vi "rad_Button and Menu Status.vi"(9 "Manager Permissions":bool, 10 "App Image List":i32, 11 "Target List":i32[](array[numeric])) -> (0 "Retrieve AppImage":bool, 1 "Deploy AppImage":bool, 2 "View Target Info":bool, 3 "Configure App Image":bool, 4 "Compare":bool, 5 "Configure Target":bool)   [LabVIEW 2013]
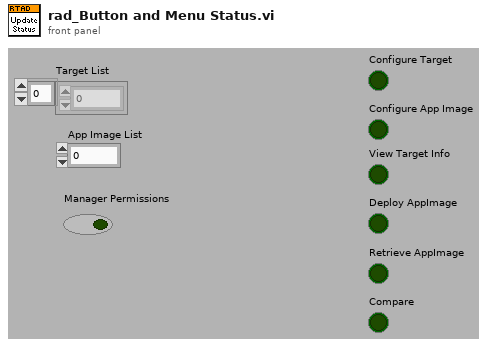
[diagram p1: front panel]
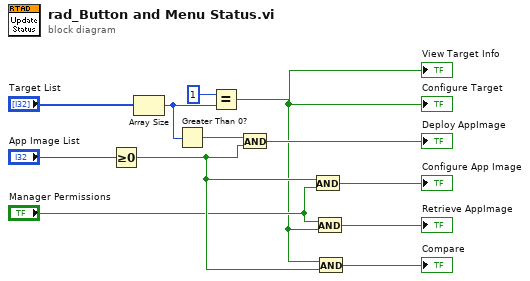
[diagram p0: block diagram]
diagram:
  n1 = Greater Or Equal To 0?(x="App Image List") -> (x >= 0?=w5:bool)
  n2 = Array Size(array="Target List") -> (size(s)=w10:i32)
  n3 = Greater Than 0?(x=w10) -> (x > 0?=w12:bool)
  n4 = Equal?(x=1, y=w10) -> (x = y?=w2:bool)
  "Configure Target" <- w2
  "View Target Info" <- w2
  n5 = And(x=w12, y=w5) -> (x .and. y?=→"Deploy AppImage":bool)
  n6 = And(x=w5, y="Manager Permissions") -> (x .and. y?=→"Configure App Image":bool)
  n7 = And(x="Manager Permissions", y=w2) -> (x .and. y?=→"Retrieve AppImage":bool)
  n8 = And(x=w2, y=w5) -> (x .and. y?=→"Compare":bool)
